vi "Timer_HasPeriodPassedOnce.vi"(8 "Pass_Through_Time":dbl=-1.0 format="%33.4f", 9 "Period":dbl, 11 "in Timer":T1 {"Accumulated TIme" format="%13.5p"; "StartTime" format="%13.5p"}) -> (1 "Expired":bool, 2 "CurrentTImer":dbl, 3 "out Timer":T1 {"Accumulated TIme" format="%13.5p"; "StartTime" format="%13.5p"})   [LabVIEW 2019, in "Trajectory_Library.lvlib"]
doc: "Check if the period specified has passed and if it has, the timer is stopped and reset. This is useful for timers that have to be timers that have to be specifically re-started after they have expired.\n\nInputs:\n - Timer -- The Timer data cluster\n - period -- The period to check for (in seconds).\n\nOutputs:\n - Timer -- The modified Timer data cluster\n - CurrentTimer -- Current time value for this timer in seconds\n - Expired -- True if the period has passed."
uses:
  Trajectory_Library.lvlib
  TypeDef/TIMER.ctl
  Util_GetTime.vi
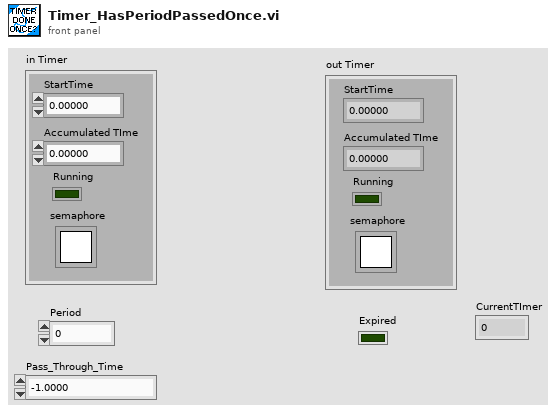
[diagram p1: front panel]
types:
  T1 = typedef "Trajectory_Library.lvlib/TIMER.ctl" = cluster{"StartTime":dbl, "Accumulated TIme":dbl, "Running":bool, "semaphore":T2}
  T2 = typedef "Semaphore RefNum" = refnum<k1>
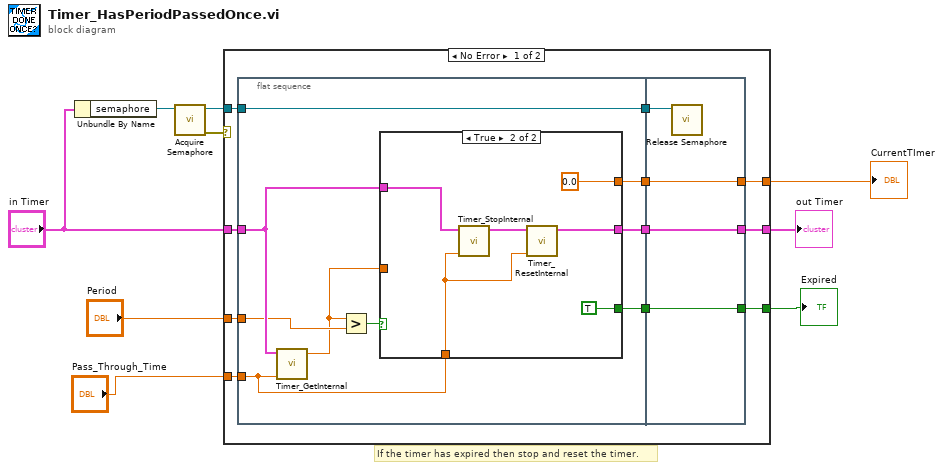
[diagram p0: block diagram]
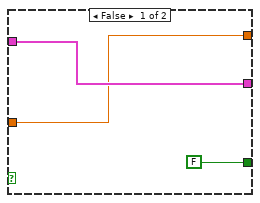
[diagram p2: hidden frame]
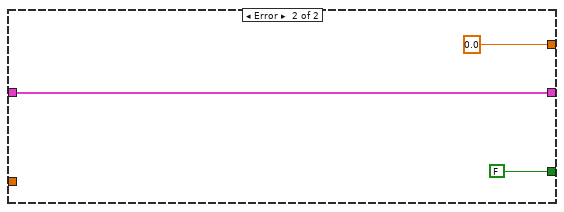
[diagram p3: hidden frame]
diagram:
  # "If the timer has expired then stop and reset the timer."
  n1 = Unbundle By Name("in Timer") -> ("semaphore"=w5:T2)
  n2 = call <vilib>:"Acquire Semaphore.vi"("semaphore"=w5) -> ("error out"=w4:errorcluster, "semaphore out"=w3:T2)  [unwired: 4 in, 1 out]
  n3 = case shown="No Error" w4 {
    tunnel: "in Timer" -> [w20 w45]
    tunnel: [w19 w45] -> w9
    tunnel: [w18 FALSE] -> w8
    tunnel: "Period" -> [w17 _]
    tunnel: w3 -> [w11 _]
    tunnel: [w16 0.0] -> w2
    tunnel: "Pass_Through_Time" -> [w10 _]
    frame No Error {
      n4 = flat-sequence {
        tunnel: w20 -> [w28]
        tunnel: w17 -> [w25]
        tunnel: [w27] -> w15
        tunnel: [w26] -> w14
        tunnel: [w23] -> w13
        tunnel: [w22] -> w12
        tunnel: w11 -> [w22]
        tunnel: w10 -> [w21]
        tunnel: [w40] -> w16
        tunnel: [w41] -> w18
        tunnel: [w42] -> w19
        tunnel: w15 -> [w42]
        tunnel: w14 -> [w41]
        tunnel: w13 -> [w40]
        tunnel: w12 -> [w39]
        frame #0 {
          n5 = call "Timer_GetInternal.vi"("Pass_Through_Time"=w21, "TIMER"=w28) -> ("CurrentTImer"=w24:dbl)  [unwired: 8 in, 1 out]
          n6 = Greater?(x=w24, y=w25) -> (0:w29:bool)
          n7 = case shown="True" w29 {
            tunnel: w28 -> [w32 w34]
            tunnel: [w32 w36] -> w27
            tunnel: [FALSE TRUE] -> w26
            tunnel: w24 -> [w30 _]
            tunnel: [w30 0.0] -> w23
            tunnel: w21 -> [_ w33]
            frame False {
            }
            frame True {
              n8 = call "Timer_StopInternal.vi"("Pass_Through_Time"=w33, "in Timer"=w34) -> ("out Timer"=w35:T1)  [unwired: 9 in]
              n9 = call "Timer_ResetInternal.vi"("Pass_Through_Time"=w33, "in TIMER"=w35) -> ("out TIMER"=w36:T1)  [unwired: 9 in]
            }
          }
        }
        frame #1 {
          n10 = call <vilib>:"Release Semaphore.vi"("semaphore"=w39) -> ()  [unwired: 5 in, 2 out]
        }
      }
    }
    frame Error {
    }
  }
  "out Timer" <- w9
  "Expired" <- w8
  "CurrentTImer" <- w2
